vi "DataLog Rotate To Chronological.vi"(7 "aggregation entries in":T1[](array[typedef]) {"point"."value" format="%.3e"; "point"."time" format="%<%H:%M:%S%2u\n%Y/%m/%d>T"}, 11 "error in (no error)":errorcluster) -> (8 "aggregation entries out":T1[](array[typedef]) {"point"."value" format="%.3e"; "point"."time" format="%<%H:%M:%S%2u\n%Y/%m/%d>T"}, 15 "dup error":errorcluster)   [LabVIEW 2012]
doc: "Rotate the recovered aggregation entries array such that it is organized in write order, first written first, last written last (with wrap gap entries at the end)."
uses:
  typedefs/clusters/t_DataLog Aggregation Entry.ctl
  typedefs/clusters/t_DataLog Point.ctl
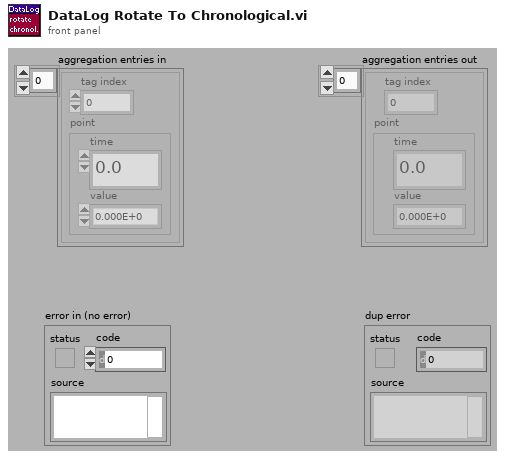
[diagram p1: front panel]
types:
  T1 = typedef "t_DataLog Aggregation Entry.ctl" = cluster{"tag index":i32, "point":T2}
  T2 = typedef "t_DataLog Point.ctl" = cluster{"time":dbl, "value":dbl}
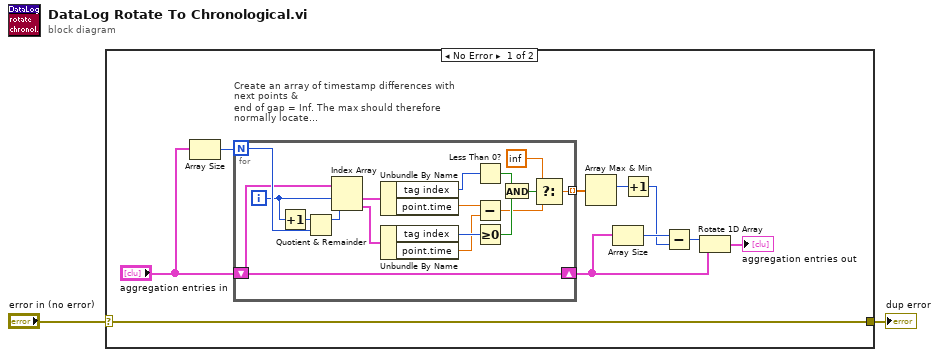
[diagram p0: block diagram]
diagram:
  n1 = case shown="No Error" "error in (no error)" {
    selector: "error in (no error)" -> [w12 w30]
    tunnel: [w12 w30] -> w2
    frame No Error {
      n2 = Array Size(array="aggregation entries in") -> (size(s)=w11:i32)
      n3 = for "Create an array of timestamp differences with next points &\nend of gap = Inf. The max should therefore normally locate\nthe end of the gap, but when the recovery file update\ncould not complete, we'll get a good shot at locating the\nwrapping point nevertheless." {
        N: w11 -> [w18]
        tunnel: [w19] -> w10 mode=indexing
        shift-right: [w15] -> w7
        shift-left: "aggregation entries in" -> [w15]
        i -> [w17]
        n4 = Increment(x=w17) -> (x+1=w16:i32)
        n5 = Quotient & Remainder(x=w16, y=w18) -> (x-y*floor(x/y)=w29:i32)  [unwired: 1 out]
        n6 = Index Array(array=w15, index #1=w17, index #2=w29) -> (element #1=w27:T1, element #2=w28:T1)
        n7 = Unbundle By Name(w27) -> ("tag index"=w26:i32, "point.time"=w14:dbl)
        n8 = Unbundle By Name(w28) -> ("tag index"=w25:i32, "point.time"=w13:dbl)
        n9 = Less Than 0?(x=w26) -> (x < 0?=w23:bool)
        n10 = Subtract(x=w14, y=w13) -> (x-y=w22:dbl)
        n11 = Greater Or Equal To 0?(x=w25) -> (x >= 0?=w24:bool)
        n12 = And(x=w23, y=w24) -> (x .and. y?=w21:bool)
        n13 = Select(t=inf, s=w21, f=w22) -> (s? t:f=w19:dbl)
      }
      n14 = Array Max & Min(array=w10) -> (max index (indices)=w9:i32)  [unwired: 3 out]
      n15 = Array Size(array=w7) -> (size(s)=w5:i32)
      n16 = Increment(x=w9) -> (x+1=w4:i32)
      n17 = Subtract(x=w5, y=w4) -> (x-y=w3:i32)
      n18 = Rotate 1D Array(1:w7, 2:w3) -> (0:→"aggregation entries out":T1[])
    }
    frame Error {
    }
  }
  "dup error" <- w2
